vi "Special_Processing.vi"(6 "cluster in":T1, 8 "error in (no error)":errorcluster, 9 "Terminal Map In":map{string, T3}(c390), 10 "Wires":T2[](array[typedef]), 11 "GrowableObjectFunction in":refnum<class "PropertyNode.lvclass">) -> (0 "error out":errorcluster, 1 "Terminal Map Out":map{string, T3}(c390), 2 "Wires out":T2[](array[typedef]), 3 "GrowableObjectFunction out":refnum<class "PropertyNode.lvclass">)   [LabVIEW 2025, in "PropertyNode.lvclass"]
uses:
  PropertyNode.lvclass
  Controls/wire.ctl
  Controls/Terminal.ctl
  Controls/bd.ctl
  Node.lvclass
  Node.lvclass/Node.ctl
  GrowableFunction.lvclass
  PropertyNode.lvclass/PropertyNode.ctl
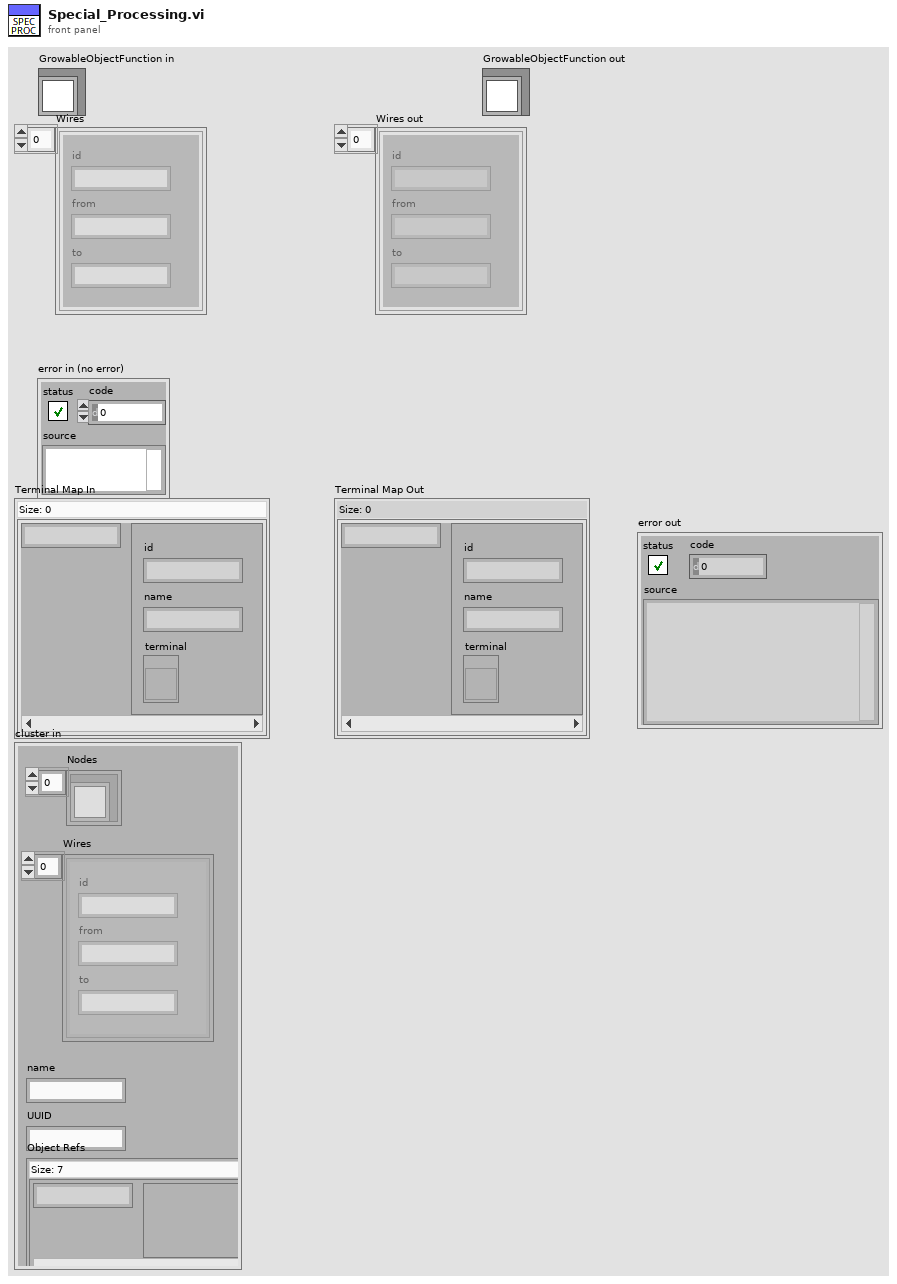
[diagram p1: front panel]
types:
  T1 = typedef "bd.ctl" = cluster{"Nodes":refnum<class "Node.lvclass">[], "Wires":T2[], "name":string, "UUID":string, "Object Refs":map{string, variant}}
  T2 = typedef "wire.ctl" = cluster{"id":string, "from":string, "to":string}
  T3 = typedef "Terminal.ctl" = cluster{"id":string, "name":string, "terminal":refnum<vi>}
  T4 = typedef "GrowableFunctionNode.ctl" = cluster{"terminalUUID":string, "Write":bool}
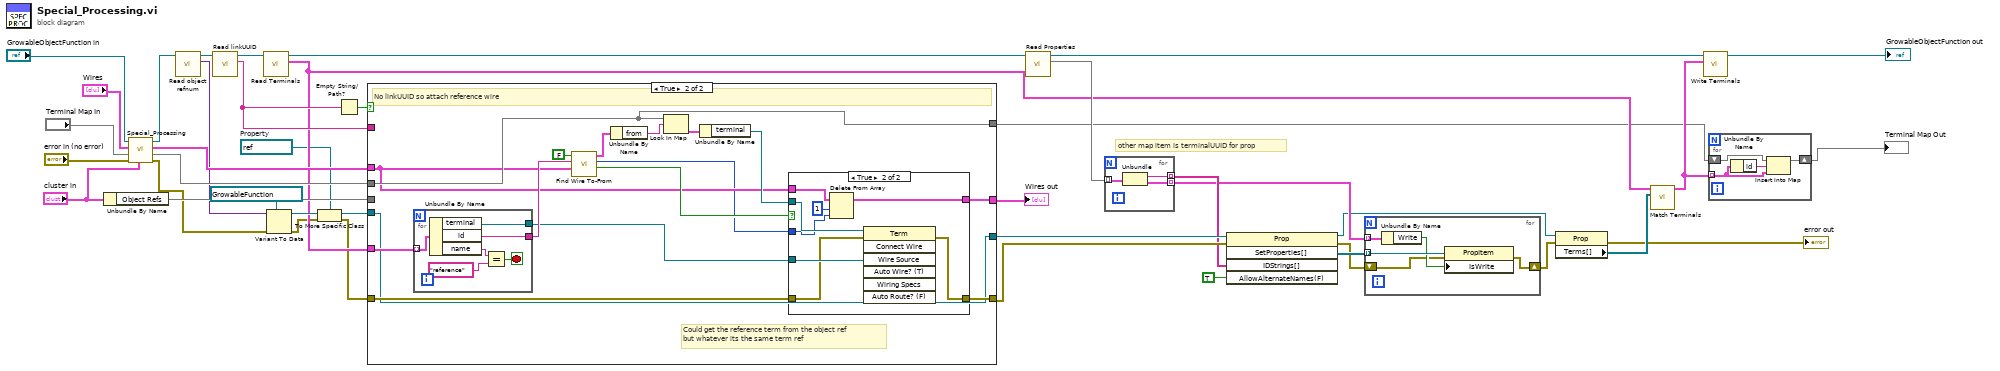
[diagram p0: block diagram]
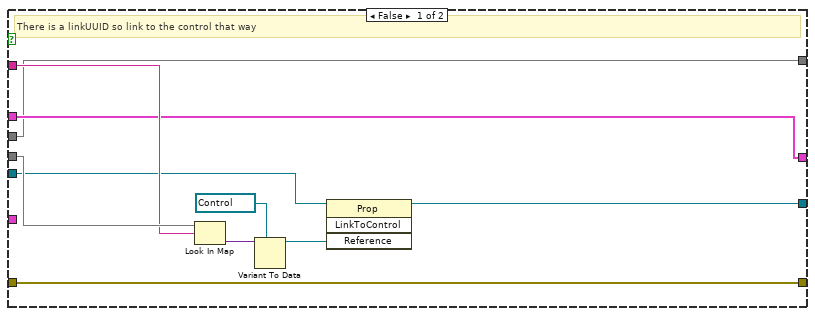
[diagram p2: hidden frame]
diagram:
  w4 = refnum<vi> refnum  # Property
  # "other map item is terminalUUID for prop"
  n1 = Unbundle By Name("cluster in") -> ("Object Refs"=w33:map{string, variant})
  n2 = call-parent "Special_Processing.vi"("cluster in"="cluster in", "error in (no error)"="error in (no error)", "Terminal Map In"="Terminal Map In", "Wires"="Wires", "Node in"="GrowableObjectFunction in") -> ("error out"=w3:errorcluster, "Terminal Map Out"=w27:map{string, T3}, "Wires out"=w30:T2[], "Node out"=w41:refnum<class "PropertyNode.lvclass">)  [unwired: 3 in]
  n3 = call-dynamic "Read object refnum.vi"("Node in"=w41) -> ("object refnum"=w23:variant, "Node out"=w36:refnum<class "PropertyNode.lvclass">)  [unwired: 8 in, 1 out]
  n4 = call-dynamic "Read linkUUID.vi"("GrowableObjectFunction in"=w36) -> ("linkUUID"=w32:string, "GrowableObjectFunction out"=w35:refnum<class "PropertyNode.lvclass">)  [unwired: 8 in, 1 out]
  n5 = call "Read Terminals.vi"("Node in"=w35) -> ("Terminals"=w17:T3[], "Node out"=w29:refnum<class "PropertyNode.lvclass">)  [unwired: 8 in, 1 out]
  n6 = Variant To Data(error in=w3, type=refnum<vi> refnum ("reference"), Variant=w23) -> (data=w24:refnum<vi>, error out=w2:errorcluster)
  n7 = To More Specific Class(target class=w4, reference=w24, error in=w2) -> (specific class reference=w5:refnum<vi>, error out=w1:errorcluster)
  n8 = Empty String/Path?(string/path=w32) -> (empty?=w34:bool)
  n9 = case shown="True" w34 {
    tunnel: w33 -> [w51 _]
    tunnel: w32 -> [w50 _]
    tunnel: w30 -> [w46 w54]
    tunnel: w17 -> [_ w67]
    tunnel: [w46 w52] -> w28
    tunnel: w27 -> [w44 w57]
    tunnel: w1 -> [w45 w59]
    tunnel: [w45 w58] -> w21
    tunnel: [w44 w57] -> w12
    tunnel: w5 -> [w43 w56]
    tunnel: [w42 w56] -> w22
    frame False {
      # "There is a linkUUID so link to the control that way"
      n10 = Look In Map(map=w51, key=w50) -> (value=w49:variant)  [unwired: 1 in, 1 out]
      n11 = Variant To Data(type=refnum<vi> refnum ("Reference"), Variant=w49) -> (data=w47:refnum<vi>)  [unwired: 1 in, 1 out]
      n12 = invoke class="Prop" method="LinkToControl"(reference=w43, "Reference"=w47) -> (reference out=w42:refnum<vi>)  [unwired: 2 in, 3 out]
    }
    frame True {
      # "Could get the reference term from the object ref \nbut whatever its the same term ref"
      # "No linkUUID so attach reference wire"
      n13 = for {
        tunnel: w67 -> [w83] mode=indexing
        tunnel: [w79] -> w66
        tunnel: [w78] -> w60
        stop <- w80 stop-if-true
        n14 = Unbundle By Name(w83) -> ("terminal"=w78:refnum<vi>, "id"=w79:string, "name"=w82:string)
        n15 = Equal?(x=w82, y="reference") -> (x = y?=w80:bool)
      }
      n16 = call "Find Wire To-From.vi"("Wires"=w54, "termUUID"=w66, "From UUID?"=FALSE) -> ("Found"=w55:bool, "Index"=w53:i32, "Wire"=w64:T2)  [unwired: 6 in]
      n17 = Unbundle By Name(w64) -> ("from"=w63:string)
      n18 = Look In Map(map=w57, key=w63) -> (value=w62:T3)  [unwired: 1 in, 1 out]
      n19 = Unbundle By Name(w62) -> ("terminal"=w61:refnum<vi>)
      n20 = case shown="True" w55 {
        tunnel: w61 -> [_ w77]
        tunnel: w60 -> [_ w76]
        tunnel: w59 -> [w69 w75]
        tunnel: [w69 w74] -> w58
        tunnel: w54 -> [w68 w73]
        tunnel: w53 -> [_ w71]
        tunnel: [w68 w70] -> w52
        frame False {
        }
        frame True {
          n21 = Delete From Array(array=w73, length=1, index=w71) -> (array with subset deleted=w70:T2[])  [unwired: 1 out]
          n22 = invoke class="Term" method="Connect Wire"(reference=w77, error in=w75, "Wire Source"=w76) -> (error out=w74:errorcluster)  [unwired: 4 in, 6 out]
        }
      }
    }
  }
  "Wires out" <- w28
  n23 = call-dynamic "Read Properties.vi"("PropertyNode in"=w29) -> ("Properties"=w20:map{string, T4}, "PropertyNode out"=w26:refnum<class "PropertyNode.lvclass">)  [unwired: 8 in, 1 out]
  n24 = for {
    tunnel: w20 -> [w86] mode=indexing
    tunnel: [w85] -> w19 mode=indexing
    tunnel: [w84] -> w9 mode=indexing
    n25 = Unbundle(w86) -> (w85:string, "GrowableFunctionNode"=w84:T4)
  }
  n26 = invoke class="Prop" method="SetProperties[]"(reference=w22, error in=w21, "IDStrings[]"=w19, "AllowAlternateNames(F)"=TRUE ("Allow Alternate Names? (F)")) -> (reference out=w8:refnum<vi>, error out=w7:errorcluster, "SetProperties[]"=w10:refnum<vi>[])  [unwired: 1 in, 2 out]
  n27 = for {
    tunnel: w10 -> [w91] mode=indexing
    tunnel: w9 -> [w90] mode=indexing
    shift-right: [w87] -> w6
    shift-left: w7 -> [w88]
    n28 = Unbundle By Name(w90) -> ("Write"=w89:bool)
    n29 = property class="PropItem"(reference=w91, error in=w88, "IsWrite"=w89) -> (error out=w87:errorcluster)  [unwired: 1 out]
  }
  n30 = property class="Prop"(reference=w8, error in=w6) -> (error out=→"error out":errorcluster, "Terms[]"=w16:refnum<vi>[])  [unwired: 1 out]
  n31 = call "Match Terminals.vi"("Terms[]"=w16, "Terminals"=w17) -> ("Terminals Out"=w13:T3[])  [unwired: 9 in]
  n32 = call "Write Terminals.vi"("Terminals"=w13, "Node in"=w26) -> ("Node out"=→"GrowableObjectFunction out":refnum<class "PropertyNode.lvclass">)  [unwired: 8 in, 1 out]
  n33 = for {
    shift-right: [w94] -> w11
    shift-left: w12 -> [w95]
    tunnel: w13 -> [w93] mode=indexing
    n34 = Unbundle By Name(w93) -> ("id"=w92:string)
    n35 = Insert Into Map(map in=w95, key=w92, value=w93) -> (map out=w94:map{string, T3})  [unwired: 2 out]
  }
  "Terminal Map Out" <- w11
